vi "Actual Temp Setpoint--SubVI.vi"(4 "Instance(1)":i32=1, 6 "Temp Setpoint Data":T1, 8 "error in (no error)":errorcluster, 11 "Watlow F4T In":refnum<class "Watlow F4T.lvclass">) -> (0 "error out":errorcluster, 2 "Actual Temp Setpoint":dbl, 3 "Watlow F4T out":refnum<class "Watlow F4T.lvclass">)   [LabVIEW 2024, in "Watlow F4T.lvclass"]
uses:
  Watlow F4T.lvclass
  Process Controller/Controls/Temp Data--Cluster.ctl
  Process Controller/Controls/Temperature Units--Enum.ctl
  Private/Controls/Standard Bus Commands--Enum.ctl
  Process Controller/_Thermal Process Controller.lvclass
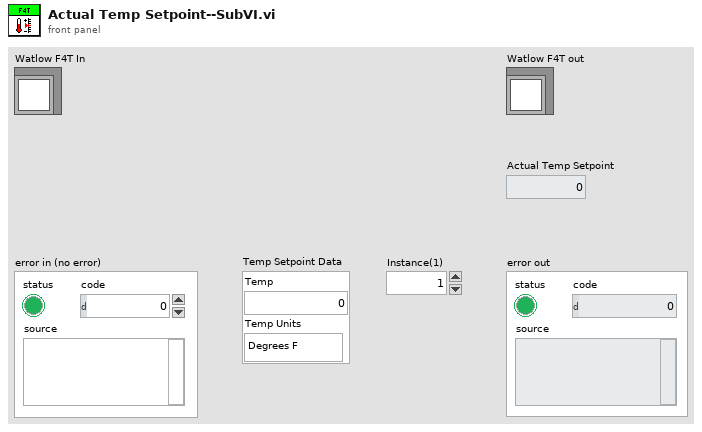
[diagram p1: front panel]
types:
  T1 = typedef "_Thermal Process Controller.lvclass/Temp Data--Cluster.ctl" = cluster{"Temp":dbl, "Temp Units":T2}
  T2 = typedef "_Thermal Process Controller.lvclass/Temperature Units--Enum.ctl" = enum16{"Degrees F", "Degrees C", "Degrees K"}
  T3 = typedef "Watlow F4T.lvclass/Standard Bus Commands--Enum.ctl" = enum16{"Remote Setpoint", "Remote Mode", "Temp Feedback", "Target Setpoint", "Current Setpoint", "Setpoint Lower Limit", "Setpoint Upper Limit", "Ramp Rate Y", "Ramp Rate X", "Ramp Rate Action", "Temp Control State", "Temp Control Mode", "Power", "Heat Power", "Cool Power"}
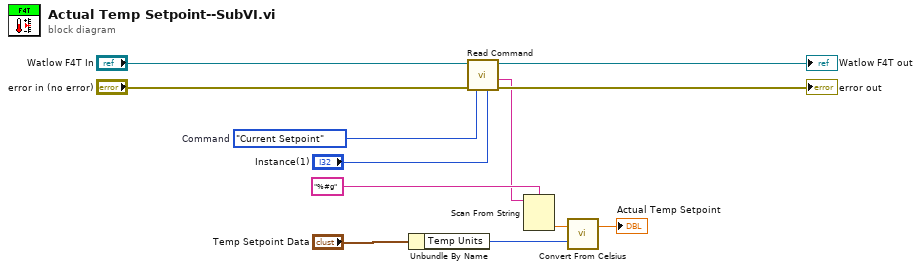
[diagram p0: block diagram]
diagram:
  w8 = Standard_Bus_Commands--Enum."Current Setpoint"  # Command
  n1 = Unbundle By Name("Temp Setpoint Data") -> ("Temp Units"=w1:T2)
  n2 = call "Read Command.vi"("Instance"="Instance(1)", "Commands"=w8, "error in (no error)"="error in (no error)", "Watlow F4T In"="Watlow F4T In") -> ("error out"=→"error out":errorcluster, "Value Out"=w4:string, "Watlow F4T out"=→"Watlow F4T out":refnum<class "Watlow F4T.lvclass">)  [unwired: 5 in]
  n3 = Scan From String(format string="%#g", input string=w4) -> (output 1=w3:dbl)  [unwired: 3 in, 3 out]
  n4 = call "Convert From Celsius.vi"("Temp In"=w3, "Temp Units"=w1) -> ("Temp Out"=→"Actual Temp Setpoint":dbl)  [unwired: 3 in]
